vi "Move Steps.vi"(8 "error in (no error)":errorcluster, 9 "Number Of Steps":T1, 10 "Model in":refnum<class "Model.lvclass">, 11 "Manual State in":refnum<class "Manual State.lvclass">) -> (0 "error out":errorcluster, 2 "Model out":refnum<class "Model.lvclass">, 3 "Manual State out":refnum<class "Manual State.lvclass">)   [LabVIEW 2016, in "Manual State.lvclass"]
uses:
  Manual State.lvclass
  Model/Model/Model.lvclass
  Typedefs/Number Of Steps.ctl
  Typedefs/HPMT_Typedefs.lvlib
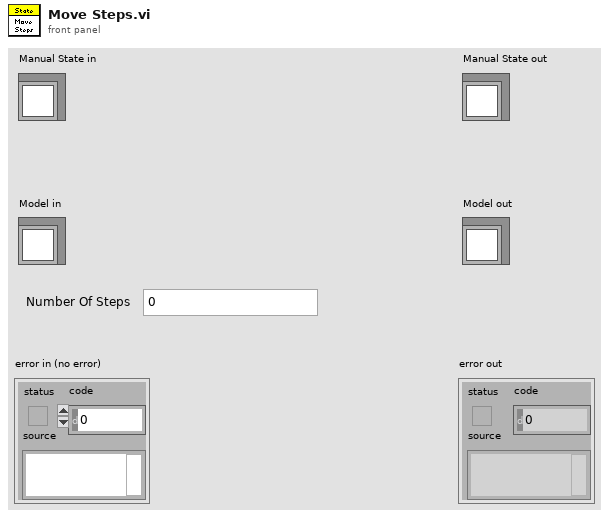
[diagram p1: front panel]
types:
  T1 = typedef "HPMT_Typedefs.lvlib/Number Of Steps.ctl" = i8
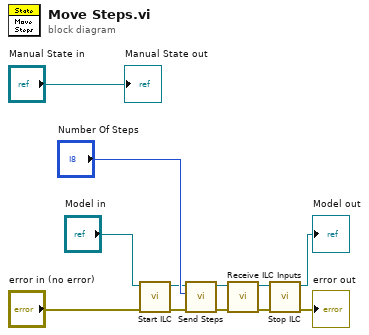
[diagram p0: block diagram]
diagram:
  n1 = call "Start ILC.vi"("error in (no error)"="error in (no error)", "Model in"="Model in") -> ("error out"=w5:errorcluster, "Model out"=w7:refnum<class "Model.lvclass">)  [unwired: 8 in]
  n2 = call "Send Steps.vi"("error in (no error)"=w5, "Command.Steps"="Number Of Steps", "Model in"=w7) -> ("error out"=w9:errorcluster, "Model out"=w10:refnum<class "Model.lvclass">)  [unwired: 7 in]
  n3 = call "Receive ILC Inputs.vi"("error in (no error)"=w9, "Model in"=w10) -> ("error out"=w2:errorcluster, "Model out"=w4:refnum<class "Model.lvclass">)  [unwired: 8 in]
  n4 = call "Stop ILC.vi"("error in (no error)"=w2, "Model in"=w4) -> ("error out"=→"error out":errorcluster, "Model out"=→"Model out":refnum<class "Model.lvclass">)  [unwired: 8 in]
  "Manual State out" <- "Manual State in"
